vi "DestroyLogger.vi"(8 "error in (no error)":errorcluster, 11 "Logger in":refnum<class "Logger.lvclass">) -> (0 "error out":errorcluster, 3 "Logger out":refnum<class "Logger.lvclass">)   [LabVIEW 2022 SP3, in "Logger.lvlib" / "Logger.lvclass"]
uses:
  Logger.lvclass
  Logger.lvclass/Logger.ctl
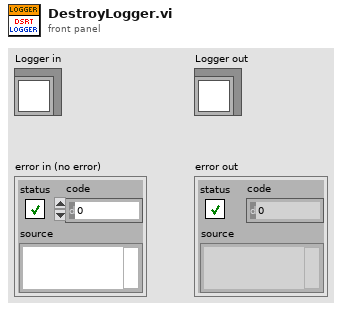
[diagram p1: front panel]
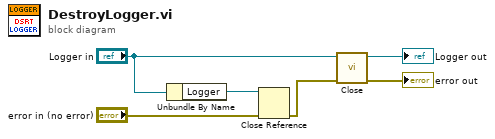
[diagram p0: block diagram]
diagram:
  n1 = Unbundle By Name("Logger in") -> ("Logger"=w3:refnum<k38>)
  n2 = Close Reference(reference=w3, error in (no error)="error in (no error)") -> (error out=w1:errorcluster)
  n3 = call-dynamic "Close.vi"("error in (no error)"=w1, "PythonWrapper in"="Logger in") -> ("error out"=→"error out":errorcluster, "PythonWrapper out"=→"Logger out":refnum<class "Logger.lvclass">)  [unwired: 8 in]
